vi "LoopScript_ChangeTime.vi"() -> ()   [LabVIEW 2017]
uses:
  CoilsControl/FrontPanelReferences.vi
  ImageAcquisitionProgram/ImageAcquisitionLibrary/GlobalFrontPanelReferences.vi
  AODControl/AODGlobals.vi
  AODControl/MessageQueue/QueueOperations/Enqueue Message (Single).vi
  CoilsControl/WaveformGenerator.lvlib
  ImageAcquisitionProgram/ImageAcquisitionLibrary/ImageAcquisitionLibrary.lvlib
  AODControl/AODControl.lvlib
  AODControl/MessageQueue/MessageQueue.lvlib
panel:
  in  "No Of Points":i32=33
  in  "Stop Between fwd/bwd":bool
  out "Current Radius":dbl
  in  "R_f":dbl
  in  "R_0":dbl
  in  "Radius Steps":i32=30
  out "Current Step Down":i32
  out "Current Step Up":i32
  out "Current Loop":i32
  in  "NumberOfLoops":i32
  in  "Record Time":u32=15000
  in  "B_f^2":dbl
  in  "B_0^2":dbl
  in  "Steps":i32=30
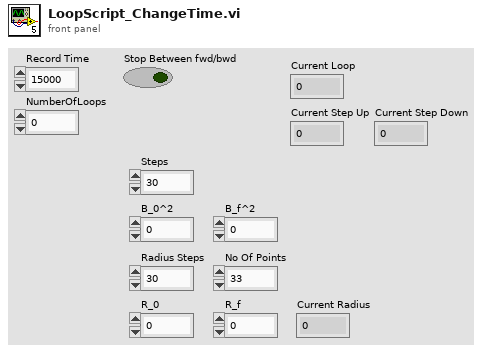
[diagram p1: front panel]
types:
  T1 = typedef "AODControl.lvlib/MessageQueue.lvlib/All Message Queues.ctl" = cluster{" AOD Interface":refnum<queue>}
  T2 = typedef "ImageAcquisitionLibrary.lvlib/References.ctl" = cluster{"Acquire":refnum<vi>, "Rec":refnum<vi>, "Tracking":refnum<vi>, "Settings":refnum<vi>, "Stop":refnum<vi>, "Initialized?":bool, "ImDisplay":refnum<vi>}
  T3 = typedef "WaveformGenerator.lvlib/WaveformGeneratorInterfaceRef.ctl" = cluster{"Waveform X":refnum<vi>, "Waveform Y":refnum<vi>, "Waveform Z":refnum<vi>, "Amplitude X":refnum<vi>, "Amplitude Y":refnum<vi>, "Amplitude Z":refnum<vi>, "Frequency X":refnum<vi>, "Frequency Y":refnum<vi>, "Frequency Z":refnum<vi>, "Phase X":refnum<vi>, "Phase Y":refnum<vi>, "Phase Z":refnum<vi>, "Offset X":refnum<vi>, "Offset Y":refnum<vi>, "Offset Z":refnum<vi>, "Stop":refnum<vi>, "On/Off":refnum<vi>, "Field^2":refnum<vi>}
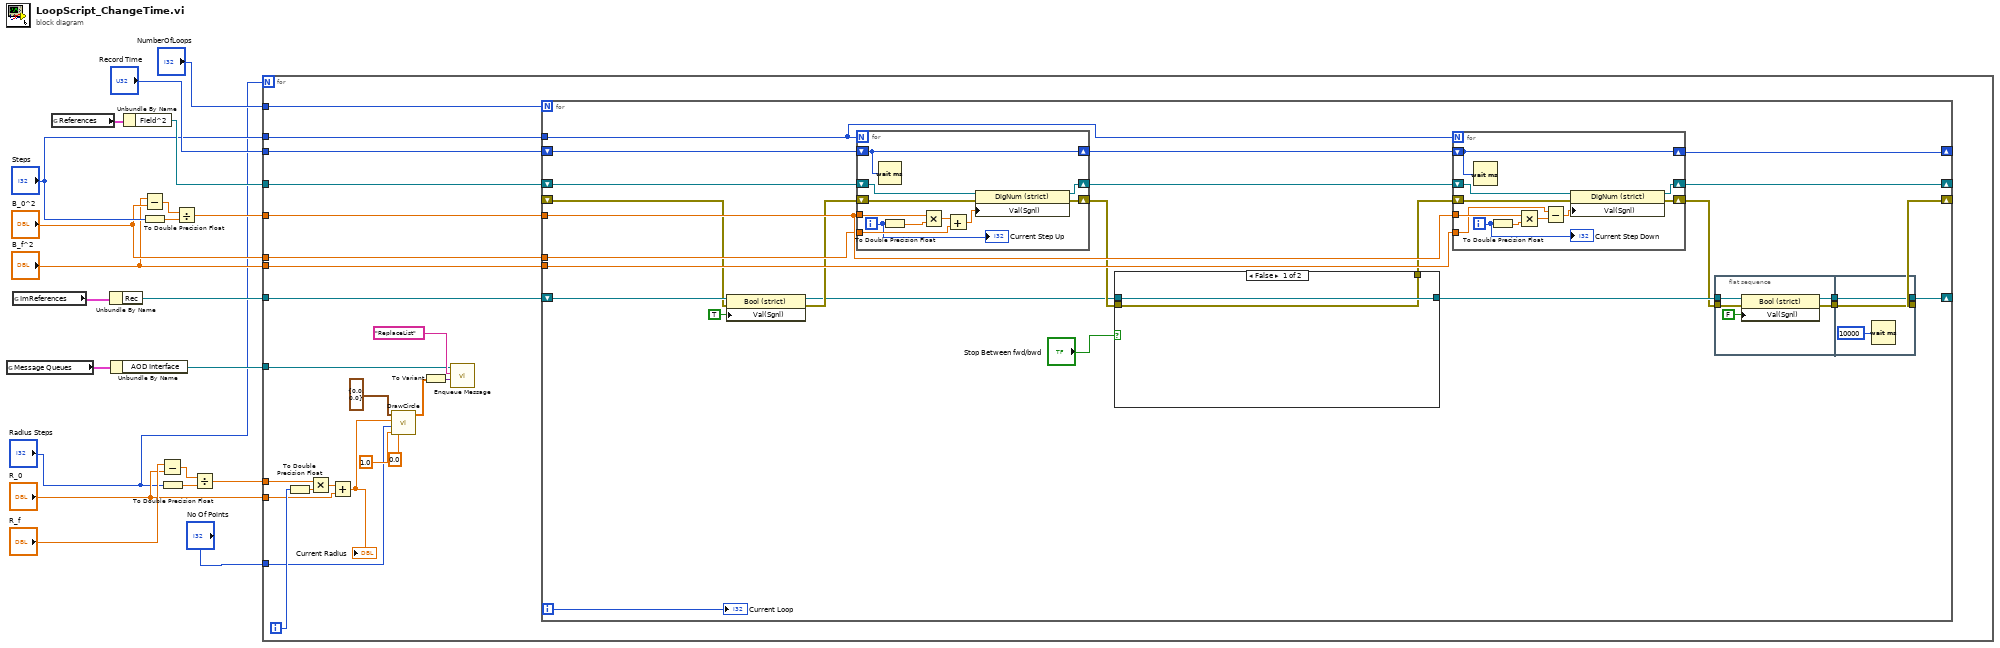
[diagram p0: block diagram]
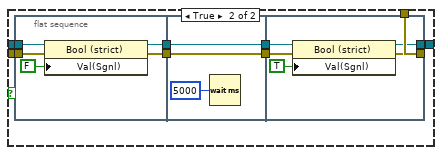
[diagram p2: hidden frame]
diagram:
  n1 = global read "AODGlobals.vi" "Message Queues"() -> (w9:T1)
  n2 = global read "GlobalFrontPanelReferences.vi" "ImReferences"() -> (w11:T2)
  n3 = global read "FrontPanelReferences.vi" "References"() -> (w21:T3)
  n4 = Unbundle By Name(w11) -> ("Rec"=w10:refnum<vi>)
  n5 = Unbundle By Name(w9) -> ("AOD Interface"=w8:refnum<queue>)
  n6 = Unbundle By Name(w21) -> ("Field^2"=w20:refnum<vi>)
  n7 = Subtract(x="B_f^2", y="B_0^2") -> (x-y=w18:dbl)
  n8 = To Double Precision Float(number="Steps") -> (double precision float=w19:dbl)
  n9 = Subtract(x="R_f", y="R_0") -> (x-y=w7:dbl)
  n10 = To Double Precision Float(number="Radius Steps") -> (double precision float=w6:dbl)
  n11 = Divide(x=w18, y=w19) -> (x/y=w15:dbl)
  n12 = Divide(x=w7, y=w6) -> (x/y=w4:dbl)
  n13 = for {
    N: "Radius Steps" -> [_]
    tunnel: w20 -> [w43]
    tunnel: "Record Time" -> [w42]
    tunnel: "Steps" -> [w41]
    tunnel: w15 -> [w40]
    tunnel: "B_0^2" -> [w39]
    tunnel: "NumberOfLoops" -> [w38]
    tunnel: "B_f^2" -> [w37]
    tunnel: w10 -> [w36]
    tunnel: w8 -> [w29]
    tunnel: w4 -> [w28]
    tunnel: "R_0" -> [w24]
    tunnel: "No Of Points" -> [w22]
    i -> [w26]
    n14 = To Double Precision Float(number=w26) -> (double precision float=w27:dbl)
    n15 = Multiply(x=w28, y=w27) -> (x*y=w25:dbl)
    n16 = Add(x=w25, y=w24) -> (x+y=w23:dbl)
    "Current Radius" <- w23
    n17 = call "DrawCircle.vi"("Phase"=0.0, "Eccentricity"=1.0, "No Of Points"=w22, "Radius"=w23, "Center"=cluster{"X":dbl, "Y":dbl} {"X"=0.0, "Y"=0.0}) -> ("Array"=w34:dbl[][])  [unwired: 6 in]
    n18 = To Variant(anything=w34) -> (Variant=w35:variant)
    n19 = call-poly "Enqueue Message.vi"("Message Data"=w35, "Message"="ReplaceList", "Message Queue"=w29) -> ()  [unwired: 7 in, 2 out]
    n20 = for {
      N: w38 -> [_]
      tunnel: w41 -> [w66]
      tunnel: w40 -> [w63]
      tunnel: w39 -> [w62]
      shift-right: [w45] -> _
      shift-left: _ -> [w49]
      shift-right: [w59] -> _
      shift-left: w43 -> [w68]
      shift-right: [w60] -> _
      shift-left: w42 -> [w67]
      tunnel: w37 -> [w58]
      shift-right: [w47] -> _
      shift-left: w36 -> [w50]
      i -> [w61]
      n21 = property class="Bool (strict)"(reference=w50, error in=w49, "Val(Sgnl)"=TRUE ("Value (Signaling)")) -> (reference out=w52:refnum<vi>, error out=w53:errorcluster)
      n22 = for {
        N: w66 -> [_]
        shift-right: [w114] -> w64
        shift-left: w68 -> [w121]
        shift-right: [w113] -> w57
        shift-left: w53 -> [w120]
        tunnel: w62 -> [w119]
        tunnel: w63 -> [w117]
        shift-right: [w112] -> w65
        shift-left: w67 -> [w112]
        i -> [w111]
        n23 = Wait (ms)(milliseconds to wait=w112) -> ()  [unwired: 1 out]
        n24 = To Double Precision Float(number=w111) -> (double precision float=w118:dbl)
        n25 = Multiply(x=w117, y=w118) -> (x*y=w116:dbl)
        n26 = Add(x=w116, y=w119) -> (x+y=w115:dbl)
        n27 = property class="DigNum (strict)"(reference=w121, error in=w120, "Val(Sgnl)"=w115) -> (reference out=w114:refnum<vi>, error out=w113:errorcluster)
        "Current Step Up" <- w111
      }
      n28 = case shown="False" "Stop Between fwd/bwd" {
        tunnel: w57 -> [w69 w74]
        tunnel: [w69 w73] -> w56
        tunnel: w52 -> [w70 w72]
        tunnel: [w70 w71] -> w48
        frame False {
        }
        frame True {
          n29 = flat-sequence {
            tunnel: w74 -> [w83]
            tunnel: w72 -> [w82]
            tunnel: [w80] -> w78
            tunnel: [w79] -> w77
            tunnel: [w85] -> w76
            tunnel: w78 -> [w85]
            tunnel: [w84] -> w75
            tunnel: w77 -> [w84]
            tunnel: w76 -> [w91]
            tunnel: w75 -> [w90]
            tunnel: [w88] -> w71
            tunnel: [w87] -> w73
            frame #0 {
              n30 = property class="Bool (strict)"(reference=w82, error in=w83, "Val(Sgnl)"=FALSE ("Value (Signaling)")) -> (reference out=w80:refnum<vi>, error out=w79:errorcluster)
            }
            frame #1 {
              n31 = Wait (ms)(milliseconds to wait=u32 5000) -> ()  [unwired: 1 out]
            }
            frame #2 {
              n32 = property class="Bool (strict)"(reference=w91, error in=w90, "Val(Sgnl)"=TRUE ("Value (Signaling)")) -> (reference out=w88:refnum<vi>, error out=w87:errorcluster)
            }
          }
        }
      }
      n33 = for {
        N: w66 -> [_]
        shift-right: [w106] -> w59
        shift-left: w64 -> [w110]
        shift-right: [w105] -> w46
        shift-left: w56 -> [w109]
        tunnel: w58 -> [w100]
        tunnel: w63 -> [w107]
        shift-right: [w104] -> w60
        shift-left: w65 -> [w104]
        i -> [w102]
        n34 = Wait (ms)(milliseconds to wait=w104) -> ()  [unwired: 1 out]
        n35 = To Double Precision Float(number=w102) -> (double precision float=w108:dbl)
        n36 = Multiply(x=w107, y=w108) -> (x*y=w101:dbl)
        n37 = Subtract(x=w100, y=w101) -> (x-y=w103:dbl)
        n38 = property class="DigNum (strict)"(reference=w110, error in=w109, "Val(Sgnl)"=w103) -> (reference out=w106:refnum<vi>, error out=w105:errorcluster)
        "Current Step Down" <- w102
      }
      n39 = flat-sequence {
        tunnel: w46 -> [w96]
        tunnel: w48 -> [w95]
        tunnel: [w93] -> w55
        tunnel: [w92] -> w54
        tunnel: w55 -> [w98]
        tunnel: w54 -> [w97]
        tunnel: [w98] -> w47
        tunnel: [w97] -> w45
        frame #0 {
          n40 = property class="Bool (strict)"(reference=w95, error in=w96, "Val(Sgnl)"=FALSE ("Value (Signaling)")) -> (reference out=w93:refnum<vi>, error out=w92:errorcluster)
        }
        frame #1 {
          n41 = Wait (ms)(milliseconds to wait=u32 10000) -> ()  [unwired: 1 out]
        }
      }
      "Current Loop" <- w61
    }
  }
